vi "Generate Gene.vi"(8 "error in":errorcluster, 11 "IGene in":refnum<class "IGene.lvclass">) -> (0 "error out":errorcluster, 3 "IGene out":refnum<class "IGene.lvclass">)   [LabVIEW 2016, in "IGene.lvclass"]
uses:
  IGene.lvclass
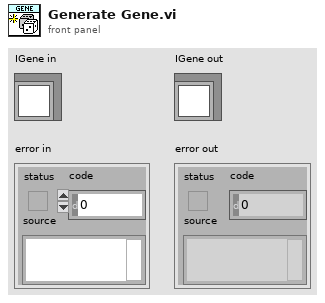
[diagram p1: front panel]
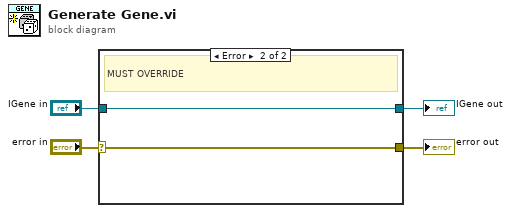
[diagram p0: block diagram]
diagram:
  n1 = case shown="Error" "error in" {
    selector: "error in" -> [w5 w8]
    tunnel: [w5 w8] -> w3
    tunnel: [w6 w7] -> w1
    tunnel: "IGene in" -> [w6 w7]
    frame No Error {
      # "MUST OVERRIDE"
    }
    frame Error {
      # "MUST OVERRIDE"
    }
  }
  "error out" <- w3
  "IGene out" <- w1
